vi "SPC_get_module_info.vi"(8 "Error In":errorcluster, 10 "Module No":i16 min=0 max=7 step=1, 11 "DLL Path":path) -> (0 "Error Out":errorcluster, 2 "Module No":i16, 3 "DLL Path":path, 5 "SPCModInfo":T1={"Module Type"=-1, "Bus Number"=0, "Slot Number"=0, "in Use"=-1, "Init Status"=-1, "Base I/O Addr"=0} {"Bus Number" min=-1 max=255 step=1; "Base I/O Addr" format="%.0x"; "Init Status" min=-10 max=0 step=1; "in Use" min=-1 max=1 step=1; "Slot Number" min=-1 max=255 step=1; "Module Type" items=["SPC-600"=600, "SPC-630"=630, "SPC-700"=700, "SPC-730"=730, "SPC-130"=130, "SPC-830"=830, "SPC-140"=140, "SPC-930"=930, "DPC-230"=230, "SPC-150"=150, "SPC-150 N"=151, "SPC-150 NX"=152, "SPC-130 EM"=131, "SPC-130 EMN"=132, "SPC-160"=160, "SPC-160 X"=161, "SPC-160 PCIE"=162, "SPC-180 N"=180, "SPC-180 NX"=181, "SPC-180 NXX"=182, "SPC-180 N-USB"=185, "SPC-180 NX-USB"=186, "SPC-180 NXX-USB"=187, "TDC-104"=104, "DPC-330"=330, "SPC-590"=590, "Simulation"=-1]})   [LabVIEW 2019]
doc: "After calling the SPC_init function the SPCModInfo internal structures for all 8 \nmodules are filled. This function transfers the contents of the internal structure of the DLL into \na structure of the type SPCModInfo (see spcm_def.h) which has to be defined by the user. The \nparameters included in this structure are described below.\nshort module_type SPC module type (see spcm_def.h)\nshort bus_number PCI bus number of the module\nshort slot_number slot number on PCI bus ‘bus_number’ occupied by the module\nshort in_use -1 used and locked by other application, 0 - not used, 1 - in use\nshort init set to initialisation result code\nunsigned short base_adr base I/O address on PCI bus\n\ninfo@becker-hickl.com"
uses:
  SPC_Controls/SPCModInfo.ctl
  SPC_Controls/ModuleType.ctl
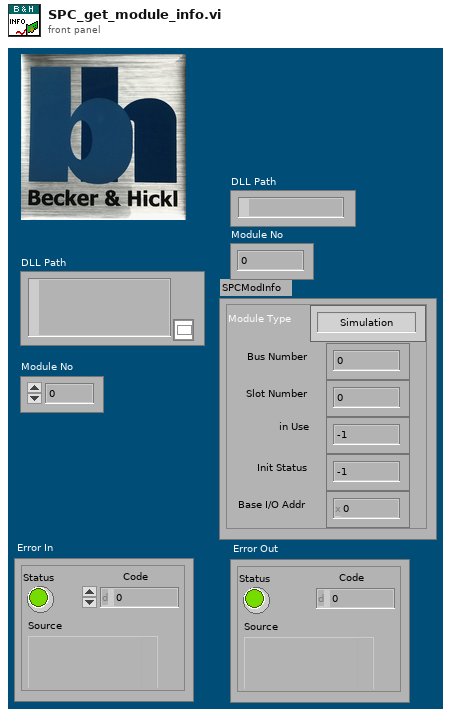
[diagram p1: front panel]
types:
  T1 = typedef "SPCModInfo.ctl" = cluster{"Module Type":T2, "Bus Number":i16, "Slot Number":i16, "in Use":i16, "Init Status":i16, "Base I/O Addr":u16}
  T2 = typedef "ModuleType.ctl" = i16
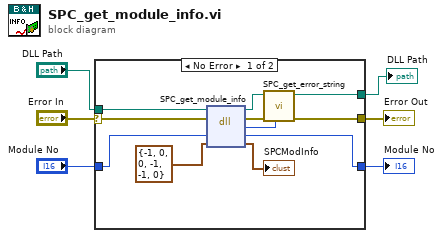
[diagram p0: block diagram]
diagram:
  n1 = case shown="No Error" "Error In" {
    selector: "Error In" -> [w15 w20]
    tunnel: "DLL Path" -> [w16 w19]
    tunnel: [w9 w19] -> w5
    tunnel: [w8 w20] -> w3
    tunnel: "Module No" -> [w13 w18]
    tunnel: [w12 w18] -> w1
    frame No Error {
      n2 = dll-call lib="D:/spcm/lib/lab_view/lv10.0/spcm32.dll" fn="SPC_get_module_info"(path in=w16, error in=w15, "mod_no"=w13, "SPC module info out"=T1 {"Module Type"=-1, "Bus Number"=0, "Slot Number"=0, "in Use"=-1, "Init Status"=-1, "Base I/O Addr"=0} ("SPC module info in")) -> (path out=w10:path, error out=w11:errorcluster, "return type"=w7:i16, "mod_no"=w12:i16, "SPC module info out"=→"SPCModInfo":T1)  [unwired: 1 in]
      n3 = call "SPC_get_error_string.vi"("ErrorID"=w7, "Error In"=w11, "DLL Path"=w10) -> ("Error Out"=w8:errorcluster, "DLL Path"=w9:path)  [unwired: 6 in, 1 out]
    }
    frame Error {
    }
  }
  "DLL Path" <- w5
  "Error Out" <- w3
  "Module No" <- w1
